vi "Dashboard Main.vi"() -> ()   [LabVIEW 2015]
uses:
  <vilib>/Utility/miscctls.llb/LVRowAndColumnTypeDef.ctl
  <vilib>/event_ctls.llb/eventvkey.ctl
  <vilib>/Rock Robotics/WPI/Dashboard/WPI_DashboardLogging Global.vi
  <vilib>/Rock Robotics/Network Tables/NT Read Numeric Array.vi
  <vilib>/Rock Robotics/Network Tables/NT Write Boolean.vi
  <vilib>/Utility/config.llb/Write Key (String).vi
  <vilib>/Utility/config.llb/Write Key (I32).vi
  <vilib>/Utility/config.llb/NI_LVConfig.lvlib
panel:
  in  "TCP":refnum<k5>
  in  "Rec Mode":enum32{"Stop", "Record", "Playback"}(radio)
  in  "Vision":u16(ring)=2 items=["Camera Off", "USB Camera SW", "USB Camera HW", "IP Camera"]
  out "Camera IP":string
  out "Image Message":string="Timeout in Camera Communications"
  in  "Dashboard Tab":T1(tab)
  in  "Select Auto":string(combo)
  out "NT Connection":bool
  in  "Camera Settings":T2={"Frame Rate"=30, "Compression"=30, "Size"=1} {"Frame Rate" scale=1.0..30.0; "Size" items=["640x480", "320x240", "160x120"]}
  out "MotorChart R":cluster{"Numeric":dbl, "Numeric":dbl}(graph)
  out "MotorChart L":T3(graph)
  out "MotorSliders R":cluster{"MotorSlide1":dbl, "MotorSlide2":dbl} {"MotorSlide2" scale=-1.0..1.0 scale format="%#_2e"; "MotorSlide1" scale=-1.0..1.0 scale format="%#_2e"}
  out "MotorSliders L":T4 {"MotorSlide4 2" scale=0.0..14.0 scale format="%#_2e"; "MotorSlide2" scale=-1.0..1.0 scale format="%#_2e"; "MotorSlide1" scale=-1.0..1.0 scale format="%#_2e"}
  out "Gyro":dbl(knob) scale=0.0..360.0
  out "JS1 Z":dbl(slide) scale=-1.0..1.0 scale format="%#_2e"
  out "JS1 Graph":cluster{"X":dbl, "Y":dbl}[](graph)
  out "JS1 Buttons":T5
  out "JS2 Z":dbl(slide) scale=-1.0..1.0 scale format="%#_2e"
  out "JS2 Graph":cluster{"X":dbl, "Y":dbl}[](graph)
  out "JS2 Buttons":T5
  out "Mode":T6(ring)=enum."Auto Disabled"
  in  "DB Camera Config":bool
  out "fps":dbl format="%#.1g"
  out "Mbps":dbl format="%#.1g"
  out "Mbps LED":bool
  in  "Camera Switch":bool
  in  "DB/String 9":string
  in  "DB/String 8":string
  in  "DB/String 7":string
  in  "DB/String 6":string
  in  "DB/String 5":string
  in  "DB/String 4":string
  in  "DB/String 3":string
  in  "DB/String 2":string
  in  "DB/String 1":string
  in  "DB/String 0":string
  in  "DB/Slider 0":dbl(slide) scale=0.0..5.0
  in  "DB/Slider 1":dbl(slide) scale=0.0..5.0
  in  "DB/Slider 2":dbl(slide) scale=0.0..5.0
  in  "DB/Slider 3":dbl(slide) scale=0.0..5.0
  out "DB/LED 3":bool
  out "DB/LED 2":bool
  out "DB/LED 1":bool
  out "DB/LED 0":bool
  in  "DB/Button 3":bool
  in  "DB/Button 2":bool
  in  "DB/Button 1":bool
  in  "DB/Button 0":bool caption="New Name"
  in  "Test Slider":dbl(slide) scale=0.0..100.0 scale format="%#_3g"
  in  "On/Off":bool caption="Solenoid"
  in  "Test Name":u16(ring) items=["Select the test to run..."]
  in  "Test Tree":string(tree)
  in  "Motor":cluster{"Value":dbl, "Enable":bool} {"Value" scale=-1.0..1.0 scale format="%#_3g"}
  out "Progress":T7 {"Test Progress" scale=0.0..100.0}
  in  "Rev/Fwd":cluster{"Forward":bool, "Reverse":bool}
  in  "Test Ring":u16(ring) items=["Monochrome", "Color"]
  out "Cmd Status":string
  in  "Execute Command":bool
  in  "Command Params":string[][](table)
  in  "Command Selection":i32(listbox)
  in  "CheckList":i32(listbox)
  out "Tree":string(tree)
  out "Camera Image":T8(plugin-control)
  out "Background":bool
  # "Left"
  # "Front"
  # "Right"
  # "Battery"
  # "This tab is a great place for autonomous settings and robot-specific values.\nPlace controls and indicators inside this tab and match name to\nDashboard Variables on robot. You can also delete this comment."
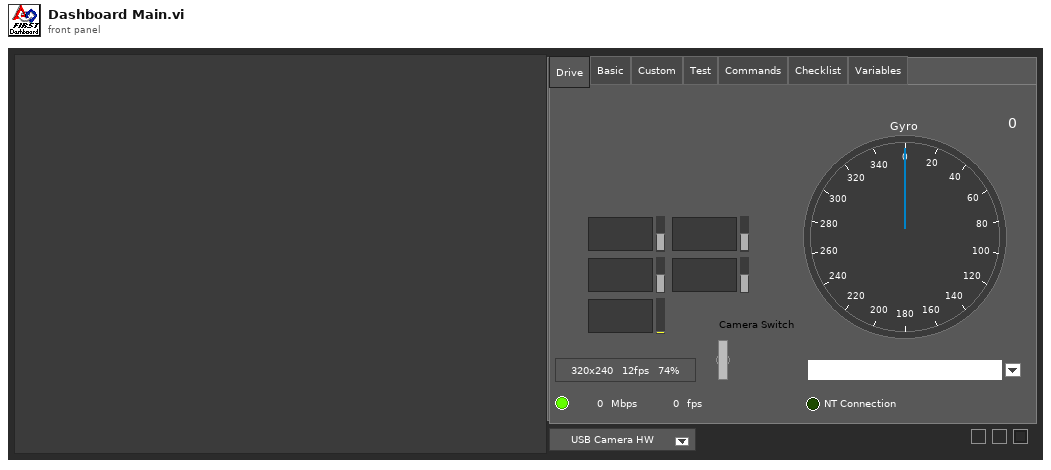
[diagram p1: front panel]
types:
  T1 = enum32{"Drive", "Basic", "Custom", "Test", "Commands", "Checklist", "Variables"}
  T2 = cluster{"Frame Rate":i32, "Compression":i32, "Size":u16}
  T3 = cluster{"Numeric":dbl, "Numeric":dbl, "Battery V":dbl}
  T4 = cluster{"MotorSlide1":dbl, "MotorSlide2":dbl, "MotorSlide4 2":dbl}
  T5 = cluster{bool, bool, bool, bool, bool, bool, bool, bool, bool, bool, bool, bool}
  T6 = enum8{"Tele-Op Disabled", "Tele-Op Enabled", "Auto Disabled", "Auto Enabled", "Test Disabled", "Test Enabled", "Disconnected", "No Code", "E-Stop"}
  T7 = cluster{"Test Progress":u8, "Test Progress Text":string}
  T8 = typedef "IMAQ Image.ctl" = refnum<image>
  T9 = cluster{"IDs":cluster{"RPC field ID":u16, "Unique ID":u16}, "String":string}
  T10 = enum32{"Drive", "Basic", "Custom", "Test", "Checklist", "Variables"}
  T11 = typedef "Image Type" = u32
  T12 = cluster{"Camera Image":refnum<vi>, "Dashboard Tab":refnum<vi>, "Background":refnum<vi>, "Vision":refnum<vi>, "Rec Mode":refnum<vi>, "Test Slider":refnum<vi>, "On/Off ":refnum<vi>, "Test Ring":refnum<vi>, "Rev/Fwd":refnum<vi>, "Test Name":refnum<vi>, "Motor":refnum<vi>, "Progress":refnum<vi>, "CheckList":refnum<vi>, "Tree":refnum<vi>, "Test Tree":refnum<vi>, "Command Params":refnum<vi>, "Command Selection":refnum<vi>, "Execute Command":refnum<vi>, "Cmd Status":refnum<vi>}
  T13 = cluster{"Error Strings":string, "Disable Counts":cluster{u16, u16}, "Rail Faults":cluster{u16, u16, u16}, "Robot IP":string, "DB Mode":u8, "Event Info":cluster{"Name":string, "Type":u8, "Number":u16, "Replay":u8}, "Camera Addr":string}
  T14 = cluster{"Storage":cluster{"Disk Free":u64, "RAM Block":u32, "RAM free":u32}, "CPU Utilization":cluster{"CPU % ISR":sgl, "CPU % Time Crit":sgl, "CPU % Timed Str":sgl, "CPU % High":sgl, "CPU % Above":sgl, "CPU % Normal":sgl, "CPU % Low":sgl}, "CAN":cluster{"% Bus Utilization":sgl, "Bus Off Cnt":u32, "TX_FIFO Full Cnt":u32, "Receive Error Cnt":u8, "Transmit Error Cnt":u8}, "HID":cluster{"HID Outputs":u32, "Rumble Low":u16, "Rumble High":u16}[]}
  T15 = cluster{"Status bits":cluster{"Test Mode":bool, "Autonomous":bool, "Enabled":bool, "Code Start":bool, "Brownout":bool, "Reserved 2":bool, "Reserved 3":bool, "E-Stop":bool}, "Code Trace":cluster{"Disabled":bool, "TeleOp":bool, "Auto":bool, "Test":bool}, "Controller Type":enum16{"unknown", "cRIO", "roboRio"}, "Code?":enum16{"unknown", "noCode", "code"}, "Battery V":dbl}
  T16 = cluster{"Control Bits":cluster{"TestMode":bool, "Autonomous":bool, "Enabled":bool, "FMS Present":bool, bool, bool, bool, "E-Stop":bool}, "Team Station ":u8, "Countdown":sgl, "Joystick Values":cluster{"Axes":dbl[], "Buttons":bool[], "POVs":i16[]}[]}
  T17 = cluster{"Axes":dbl[], "Buttons":bool[], "POVs":i16[]}[]
  T18 = cluster{"Axes":dbl[], "Buttons":bool[], "POVs":i16[]}
  T19 = cluster{"Buttons[0]":bool, "Buttons[1]":bool, "Buttons[2]":bool, "Buttons[3]":bool, "Buttons[4]":bool, "Buttons[5]":bool, "Buttons[6]":bool, "Buttons[7]":bool, "Buttons[8]":bool, "Buttons[9]":bool, "Buttons[10]":bool, "Buttons[11]":bool}
  T20 = typedef "NI_LVConfig.lvlib/Config Data RefNum.ctl" = refnum<k1>
  T21 = cluster{"Operation":enum16{"Update", "Clear"}, "Color Box":u32}[]
  T22 = typedef "eventvkey.ctl" = enum16{"ASCII", "Enter", "Return", "Shift", "Ctrl", "Alt", "Cmd", "Opt", "Caps", "NumLock", "Clear", "Break", "Up", "Down", "Left", "Right", "Insert", "Delete", "Home", "End", "PageUp", "PageDown", "Escape", "Help", "Pause", "ScrollLock", "F1", "F2", "F3", "F4", "F5", "F6", "F7", "F8", "F9", "F10", "F11", "F12", "F13", "F14", "F15", "F16", "F17", "F18", "F19", "F20", "F21", "F22", "F23", "F24", "Play", "VolumeUp", "VolumeDown", "Mute", "Two Byte Char"}
  T23 = cluster{"Image Size":bool, "Image Type":bool, "Pixel Value":bool, "ROI Information":bool, "Zoom Factor":bool}
  T24 = enum8{"Enabled", "Disabled", "Disabled and Grayed Out"}
  T25 = cluster{"Operation":enum16{"Update", "Clear"}, "Color Box":u32}
  T26 = typedef "LVRowAndColumnTypeDef.ctl" = cluster{"Row":i32, "Column":i32}
  T27 = cluster{"Shift":bool, "Ctrl":bool, "Alt":bool, "Cmd":bool, "Opt":bool}
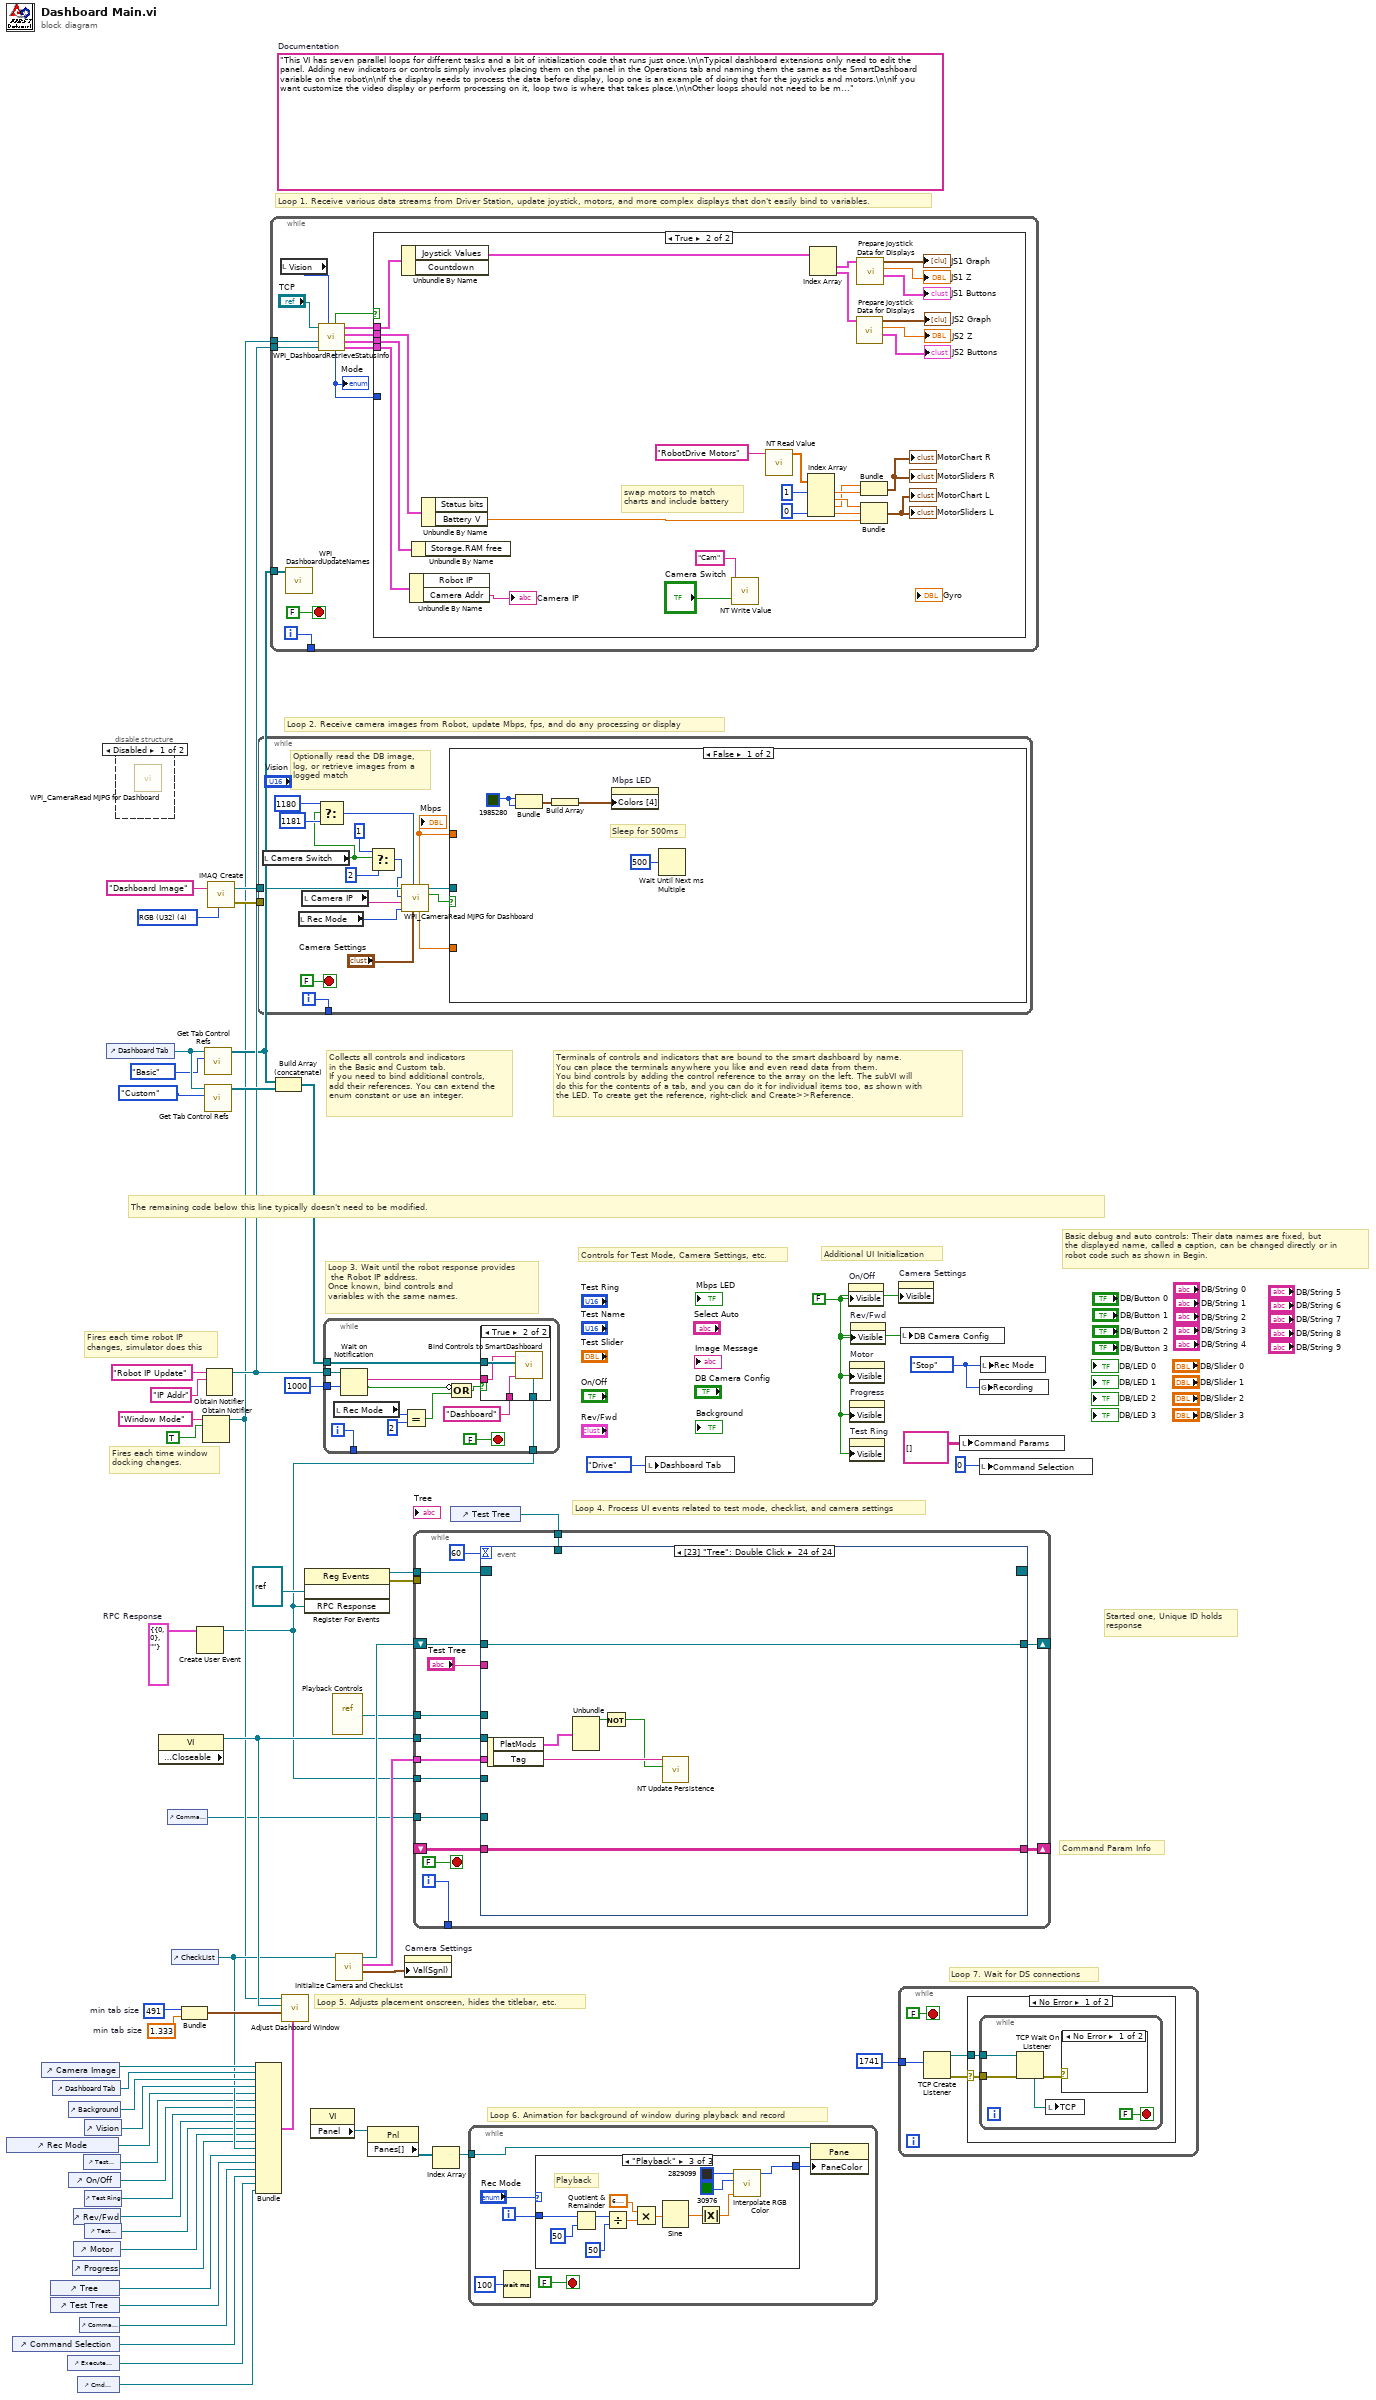
[diagram p0: block diagram]
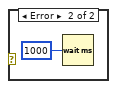
[diagram p3: hidden frame]
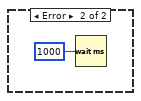
[diagram p4: hidden frame]
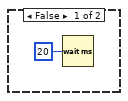
[diagram p5: hidden frame]
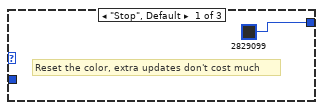
[diagram p6: hidden frame]
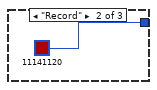
[diagram p7: hidden frame]
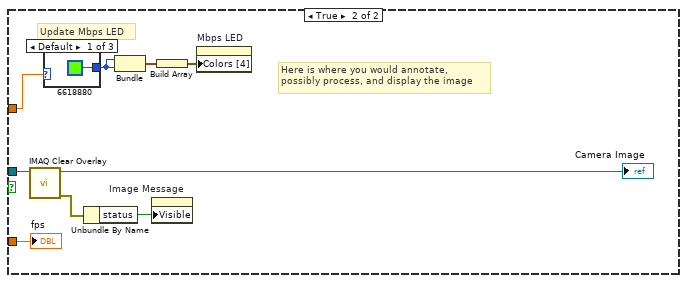
[diagram p9: hidden frame]
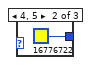
[diagram p10: hidden frame]
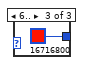
[diagram p11: hidden frame]
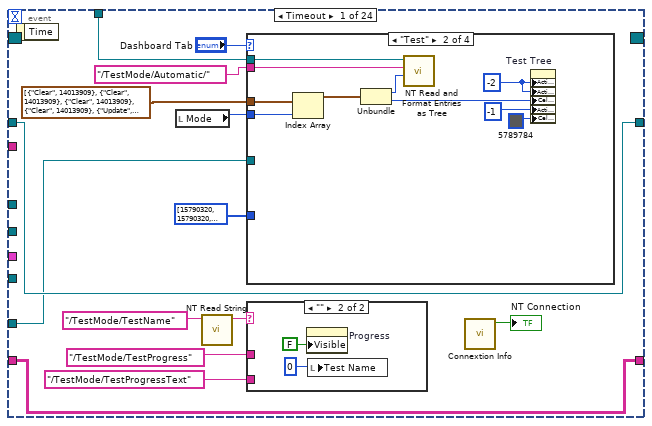
[diagram p12: hidden frame]
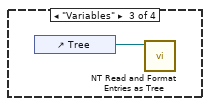
[diagram p14: hidden frame]
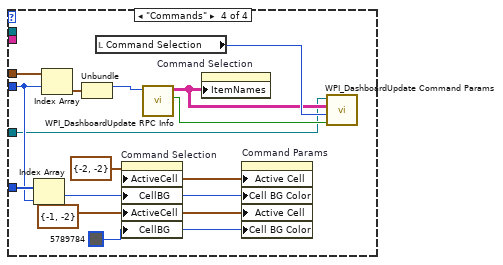
[diagram p15: hidden frame]
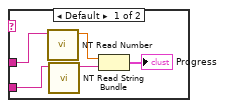
[diagram p16: hidden frame]
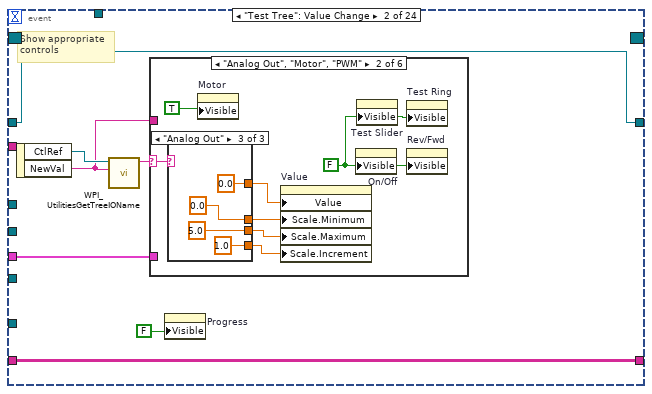
[diagram p17: hidden frame]
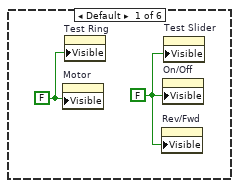
[diagram p18: hidden frame]
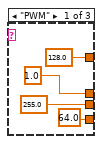
[diagram p19: hidden frame]
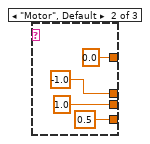
[diagram p20: hidden frame]
diagram:
  w7 = T9 {"IDs"={"RPC field ID"=0, "Unique ID"=0}, "String"=""}  # RPC Response
  w33 = 491  # min tab size
  w32 = 1.333  # min tab size
  w41 = enum32{"Stop", "Record", "Playback"}."Stop" ("Rec Mode")
  w15 = FALSE ("Visible")
  (unwired) "This VI has seven parallel loops for different tasks and a bit of initialization code that runs just once.\n\nTypical dashboard extensions only need to edit the panel. Adding new indicators or controls simply involves placing them on the panel in the Operations tab and naming them the same as the SmartDashboard variable on the robot\n\nIf the display needs to process the data before display, loop one is an example of doing that for the joysticks and motors.\n\nIf you want customize the video display or perform processing on it, loop two is where that takes place.\n\nOther loops should not need to be modified. They are pretty standard, and document the task they perform."  # Documentation
  w61 = T11 4 items=["Grayscale (U8)", "Grayscale (I16)", "Grayscale (SGL)", "Complex (CSG)", "RGB (U32)", "HSL (U32)", "RGB (U64)"] ("Image Type")
  # "Command Param Info"
  # "Started one, Unique ID holds\nresponse"
  # "Loop 7. Wait for DS connections"
  # "Basic debug and auto controls: Their data names are fixed, but\nthe displayed name, called a caption, can be changed directly or in\nrobot code such as shown in Begin."
  # "Controls for Test Mode, Camera Settings, etc."
  # "Additional UI Initialization"
  # "Loop 6. Animation for background of window during playback and record"
  # "Fires each time robot IP\nchanges, simulator does this"
  # "Fires each time window\ndocking changes."
  # "Collects all controls and indicators\nin the Basic and Custom tab.\nIf you need to bind additional controls,\nadd their references. You can extend the\nenum constant or use an integer."
  # "The remaining code below this line typically doesn't need to be modified."
  # "Loop 4. Process UI events related to test mode, checklist, and camera settings"
  # "Terminals of controls and indicators that are bound to the smart dashboard by name.\nYou can place the terminals anywhere you like and even read data from them.\nYou bind controls by adding the control reference to the array on the left. The subVI will\ndo this for the contents of a tab, and you can do it for individual items too, as shown with\nthe LED. To create get the reference, right-click and Create>>Reference."
  # "Loop 3. Wait until the robot response provides\n the Robot IP address.\nOnce known, bind controls and\nvariables with the same names."
  # "Loop 5. Adjusts placement onscreen, hides the titlebar, etc."
  # "Loop 1. Receive various data streams from Driver Station, update joystick, motors, and more complex displays that don't easily bind to variables."
  # "Loop 2. Receive camera images from Robot, update Mbps, fps, and do any processing or display"
  n1 = control-ref of="Rec Mode"() -> (w21:refnum<vi>)
  n2 = control-ref of="Command Selection"() -> (w6:refnum<vi>)
  n3 = control-ref of="Camera Image"() -> (w36:refnum<vi>)
  n4 = control-ref of="Tree"() -> (w25:refnum<vi>)
  n5 = control-ref of="Test Tree"() -> (w24:refnum<vi>)
  n6 = control-ref of="Dashboard Tab"() -> (w35:refnum<vi>)
  n7 = control-ref of="Execute Command"() -> (w8:refnum<vi>)
  n8 = control-ref of="Background"() -> (w30:refnum<vi>)
  n9 = control-ref of="On/Off"() -> (w19:refnum<vi>)
  n10 = control-ref of="Progress"() -> (w16:refnum<vi>)
  n11 = control-ref of="Rev/Fwd"() -> (w17:refnum<vi>)
  n12 = control-ref of="Motor"() -> (w22:refnum<vi>)
  n13 = control-ref of="Cmd Status"() -> (w2:refnum<vi>)
  n14 = control-ref of="Command Params"() -> (w9:refnum<vi>)
  n15 = control-ref of="Test Slider"() -> (w20:refnum<vi>)
  n16 = control-ref of="Vision"() -> (w34:refnum<vi>)
  n17 = control-ref of="Test Ring"() -> (w18:refnum<vi>)
  n18 = control-ref of="Test Name"() -> (w23:refnum<vi>)
  n19 = control-ref of="Dashboard Tab"() -> (w39:refnum<vi>)
  n20 = disable-structure shown="Disabled" {
    frame Disabled {
      n21 = call <vilib>:"WPI_CameraRead MJPG for Dashboard.vi"() -> ()  [unwired: 8 in, 4 out]
    }
    frame Enabled {
    }
  }
  n22 = property class="VI" props=["Front Panel.Closeable"]() -> (reference out=w40:refnum<vi>)  [unwired: 2 in, 2 out]
  n23 = control-ref of="Command Params"() -> (w1:refnum<vi>)
  n24 = control-ref of="CheckList"() -> (w26:refnum<vi>)
  n25 = Bundle("min tab size"=w33, "min tab size"=w32) -> (w31:cluster{"min tab size":i32, "min tab size":dbl})  [unwired: 1 in]
  n26 = Create User Event(user event datatype=w7) -> (user event=w3:refnum<user-event>)  [unwired: 1 in, 1 out]
  n27 = Obtain Notifier(name (unnamed)="Window Mode", notification data type=TRUE) -> (notifier out=w12:refnum<notifier>)  [unwired: 2 in, 2 out]
  n28 = call <vilib>:"Get Tab Control Refs.vi"("Page Index"=T10."Basic" ("Dashboard Tab"), "TabControl in"=w39) -> ("ControlsOnPage"=w13:refnum<vi>[])  [unwired: 9 in]
  n29 = call <vilib>:"Get Tab Control Refs.vi"("Page Index"=T10."Custom" ("Dashboard Tab"), "TabControl in"=w39) -> ("ControlsOnPage"=w38:refnum<vi>[])  [unwired: 9 in]
  n30 = Obtain Notifier(name (unnamed)="Robot IP Update", notification data type="IP Addr" ("name (unnamed)")) -> (notifier out=w14:refnum<notifier>)  [unwired: 2 in, 2 out]
  n31 = call "IMAQ Create"("Image Name"="Dashboard Image", "Image Type"=w61) -> ("New Image"=w59:T8, "error out"=w58:errorcluster)  [unwired: 2 in, 1 out]
  n32 = Bundle("Camera Image"=w36, "Dashboard Tab"=w35, "Background"=w30, "Vision"=w34, "Rec Mode"=w21, "Test Slider"=w20, "On/Off"=w19, "Test Ring"=w18, "Rev/Fwd"=w17, "Test Name"=w23, "Motor"=w22, "Progress"=w16, "CheckList"=w26, "Tree"=w25, "Test Tree"=w24, "Command Params"=w9, "Command Selection"=w6, "Execute Command"=w8, "Cmd Status"=w2) -> (w27:T12)  [unwired: 1 in]
  n33 = while {
    tunnel: w59 -> [w76]
    tunnel: w58 -> [_]
    tunnel: [w77] -> _
    i -> [w77]
    stop <- FALSE stop-if-true
    # "Optionally read the DB image,\nlog, or retrieve images from a\nlogged match"
    n34 = local read "Camera Switch"() -> (w65:bool)
    n35 = local read "Rec Mode"() -> (w71:enum32{"Stop", "Record", "Playback"})
    n36 = local read "Camera IP"() -> (w70:string)
    n37 = Select(t=1180, s=w65, f=1181) -> (s? t:f=w67:i32)
    n38 = Select(t=1, s=w65, f=2) -> (s? t:f=w62:i32)
    n39 = call <vilib>:"WPI_CameraRead MJPG for Dashboard.vi"("Camera Settings"="Camera Settings", "Camera Port"=w67, "Rec Mode"=w71, "Camera IP"=w70, "Camera Mode"=w62, "Refnum in"=w76) -> ("Active"=w74:bool, "Refnum out"=w75:T8, "FPS"=w73:dbl, "Bandwidth (Mbps)"=w69:dbl)  [unwired: 2 in]
    "Mbps" <- w69
    n40 = case shown="False" w74 {
      tunnel: w75 -> [_ w86]
      tunnel: w69 -> [_ w85]
      tunnel: w73 -> [_ w83]
      frame False {
        w79 = u32 1985280 ("Color Box")
        # "Sleep for 500ms"
        n41 = Bundle("Color Box"=w79, "Color Box"=w79) -> (w81:cluster{"Color Box":u32, "Color Box":u32})  [unwired: 1 out]
        n42 = Build Array(w81) -> (w80:cluster{"Color Box":u32, "Color Box":u32}[])
        n43 = property on="Mbps LED" class="Bool (strict)"("Colors [4]"=w80) -> ()  [unwired: 2 in, 2 out]
        n44 = Wait Until Next ms Multiple(millisecond multiple=u32 500) -> ()  [unwired: 1 out]
      }
      frame True {
        # "Here is where you would annotate,\npossibly process, and display the image"
        # "Update Mbps LED"
        n45 = call "IMAQ Clear Overlay"("Image"=w86) -> ("error out"=w90:errorcluster, "Image Out"=→"Camera Image":T8)  [unwired: 2 in, 7 out]
        n46 = case shown="Default" w85 {
          tunnel: [u32 6618880 ("Color Box") u32 16776722 ("Color Box") u32 16716800 ("Color Box")] -> w87
          frame Default {
          }
          frame 4, 5 {
          }
          frame 6.. {
          }
        }
        n47 = Unbundle By Name(w90) -> ("status"=w91:bool)
        n48 = Bundle("Color Box"=w87, "Color Box"=w87) -> (w89:cluster{"Color Box":u32, "Color Box":u32})  [unwired: 1 out]
        n49 = property on="Image Message" class="Str"("Visible"=w91) -> ()  [unwired: 2 in, 2 out]
        n50 = Build Array(w89) -> (w88:cluster{"Color Box":u32, "Color Box":u32}[])
        n51 = property on="Mbps LED" class="Bool (strict)"("Colors [4]"=w88) -> ()  [unwired: 2 in, 2 out]
        "fps" <- w83
      }
    }
  }
  n52 = while {
    tunnel: [w106] -> _
    tunnel: w14 -> [w100]
    tunnel: w13 -> [w99]
    tunnel: w12 -> [w95]
    i -> [w106]
    stop <- FALSE stop-if-true
    n53 = local read "Vision"() -> (w97:u16)
    n54 = call <vilib>:"WPI_DashboardUpdateNames.vi"("Controls on Tab"=w99) -> ()  [unwired: 11 in]
    n55 = call <vilib>:"WPI_DashboardRetrieveStatusInfo.vi"("Vision"=w97, "Binding Refnum"=w100, "Window Mode Notifier"=w95, "TCP Cnx"="TCP") -> ("Power and Errors"=w101:T13, "Robot Metrics"=w104:T14, "Status Info"=w105:T15, "Control Info"=w102:T16, "Robot Mode"=w98:T6, "Process?"=w103:bool)  [unwired: 2 in]
    "Mode" <- w98
    n56 = case shown="True" w103 {
      tunnel: w105 -> [_ w135]
      tunnel: w104 -> [_ w134]
      tunnel: w102 -> [_ w133]
      tunnel: w101 -> [_ w132]
      tunnel: w98 -> [_ _]
      frame False {
        n57 = Wait (ms)(milliseconds to wait=u32 20) -> ()  [unwired: 1 out]
      }
      frame True {
        # "swap motors to match\ncharts and include battery"
        n58 = Unbundle By Name(w133) -> ("Joystick Values"=w122:T17)  [unwired: 1 out]
        n59 = Unbundle By Name(w132) -> ("Camera Addr"=→"Camera IP":string)  [unwired: 1 out]
        n60 = Unbundle By Name(w134) -> ()  [unwired: 1 out]
        n61 = Unbundle By Name(w135) -> ("Battery V"=w123:dbl)  [unwired: 1 out]
        n62 = call-poly <vilib>:"NT Write Value.vi"("Boolean"="Camera Switch", "Name"="Cam") -> ()  [unwired: 9 in, 1 out]
        n63 = call-poly <vilib>:"NT Read Value.vi"("Name"="RobotDrive Motors") -> ("Numeric Array"=w111:dbl[])  [unwired: 9 in, 1 out]
        n64 = Index Array(array=w111, index #1=1, index #4=0) -> (element #1=w127:dbl, element #2=w128:dbl, element #3=w126:dbl, element #4=w131:dbl)  [unwired: 2 in]
        n65 = Index Array(array=w122) -> (element #1=w121:T18, element #2=w116:T18)  [unwired: 2 in]
        n66 = call "Prepare Joystick Data for Displays.vi"("Joystick Values"=w116) -> ("Buttons"=→"JS2 Buttons":T19, "Z Axis"=→"JS2 Z":dbl, "Cartesian Data"=→"JS2 Graph":cluster{"X axis":dbl, "X axis":dbl}[])  [unwired: 8 in]
        n67 = call "Prepare Joystick Data for Displays.vi"("Joystick Values"=w121) -> ("Buttons"=→"JS1 Buttons":T19, "Z Axis"=→"JS1 Z":dbl, "Cartesian Data"=→"JS1 Graph":cluster{"X axis":dbl, "X axis":dbl}[])  [unwired: 8 in]
        n68 = Bundle("Numeric"=w126, "Numeric"=w127) -> (→"MotorChart R" →"MotorSliders R":cluster{"Numeric":dbl, "Numeric":dbl})  [unwired: 1 in]
        n69 = Bundle("Numeric"=w128, "Numeric"=w131, "Battery V"=w123) -> (→"MotorChart L" →"MotorSliders L":T3)  [unwired: 1 in]
      }
    }
  }
  n70 = Build Array (concatenate)(w13, w38) -> (w37:refnum<vi>[])
  n71 = call "Adjust Dashboard Window.vi"("Sizing Refnums"=w27, "Size Constraints"=w31, "VI"=w40, "WIn Mode"=w12) -> ()  [unwired: 8 in]
  n72 = register-events(refnum<vi> refnum, w3) -> (reference out=w45:refnum<event-registration>, error out=w44:errorcluster)  [unwired: 2 in]
  n73 = property class="VI"() -> ("Panel"=w48:refnum<vi>)  [unwired: 2 in, 2 out]
  n74 = while {
    tunnel: w37 -> [w148]
    tunnel: w14 -> [w146]
    tunnel: [w144] -> _
    tunnel: u32 1000 ("milliseconds to wait") -> [w143]
    tunnel: w3 -> [w136]
    i -> [w144]
    stop <- FALSE stop-if-true
    n75 = local read "Rec Mode"() -> (w139:enum32{"Stop", "Record", "Playback"})
    n76 = Wait on Notification(notifier=w146, timeout in ms (-1)=w143) -> (notification=w145:string, timed out?=w141:bool)  [unwired: 2 in, 2 out]
    n77 = Equal?(x=w139, y=u16 2 ("Rec Mode")) -> (x = y?=w140:bool)
    n78 = Compound Arithmetic op=OR(invert w141, w140) -> (w142:bool)
    n79 = case shown="True" w142 {
      tunnel: w148 -> [_ w152]
      tunnel: w145 -> [_ w151]
      tunnel: "Dashboard" -> [_ w150]
      tunnel: w136 -> [_ w149]
      frame False {
      }
      frame True {
        n80 = call <vilib>:"Bind Controls to SmartDashboard.vi"("RPC ref"=w149, "Client Name"=w150, "Bound Control Refs"=w152, "Server IP Address"=w151) -> ()  [unwired: 8 in]
      }
    }
  }
  n81 = vi-ref "Playback Controls.vi"() -> (w46:refnum<vi>)
  n82 = call "Initialize Camera and CheckList.vi"("ListBox in"=w26) -> ("Cluster"=w52:cluster{"value":i32, "value":i32, "index":i32}, "Array"=w53:cluster{string[]}[], "File Refnum"=w51:T20)  [unwired: 8 in]
  n83 = property class="Pnl"(reference=w48) -> ("Panes[]"=w49:refnum<vi>[])  [unwired: 1 in, 2 out]
  n84 = property on="Camera Settings" class="Clust (strict)"("Val(Sgnl)"=w52) -> ()  [unwired: 2 in, 2 out]
  n85 = Index Array(array=w49) -> (element=w47:refnum<vi>)  [unwired: 1 in]
  n86 = control-ref of="Test Tree"() -> (w50:refnum<vi>)
  n87 = while {
    tunnel: w53 -> [w164]
    shift-right: [w163] -> _
    shift-left: w51 -> [w162]
    tunnel: [w161] -> _
    tunnel: w50 -> [w160]
    tunnel: w46 -> [w159]
    tunnel: w45 -> [w158]
    tunnel: w44 -> [_]
    tunnel: w40 -> [w157]
    tunnel: w3 -> [w156]
    tunnel: w1 -> [w155]
    shift-right: [w154] -> _
    shift-left: _ -> [w153]
    i -> [w161]
    stop <- FALSE stop-if-true
    n88 = event shown="[23] \"Tree\": Double Click" {
      selector: w158 -> [_ _ _ _ _ _ _ _ _ _ _ _ _ _ _ _ _ _ _ _ _ _ _ _]
      dyn-events: [_ _ _ _ _ _ _ _ _ _ _ _ _ _ _ _ _ _ w473 _ _ _ _ _] -> _
      timeout: u32 60 ("milliseconds to wait") -> [_ _ _ _ _ _ _ _ _ _ _ _ _ _ _ _ _ _ _ _ _ _ _ _]
      tunnel: w160 -> [w177 _ _ _ _ _ _ _ _ _ _ _ _ _ _ _ _ _ _ _ _ _ _ _]
      tunnel: "Test Tree" -> [_ _ _ _ _ _ _ _ _ _ _ _ _ w436 w445 w448 w453 w462 _ _ _ _ _ _]
      tunnel: w164 -> [_ w215 _ _ _ _ _ _ _ _ _ w398 w429 _ _ _ _ _ _ _ _ _ _ _]
      tunnel: [w174 w214 w318 w324 w334 w338 w344 w356 w364 w370 w383 w397 w422 w435 w443 w447 w452 w461 w475 w491 w493 w501 w512 w517] -> w163
      tunnel: w162 -> [w174 w214 w318 w324 w334 w338 w344 w356 w364 w370 w383 w396 w422 w435 w443 w447 w452 w461 w475 w491 w493 w501 w512 w517]
      tunnel: w159 -> [_ _ _ _ _ _ _ _ _ _ _ _ _ _ _ _ _ _ w476 _ w496 _ _ _]
      tunnel: w157 -> [_ _ _ _ _ _ _ _ _ _ _ _ _ _ _ _ _ _ w471 _ _ _ _ _]
      tunnel: w156 -> [_ _ _ _ _ _ _ _ _ _ _ _ _ _ _ _ _ _ w467 _ _ _ _ _]
      tunnel: w155 -> [w169 _ _ _ _ _ w342 _ _ _ _ _ _ _ _ _ _ _ _ _ _ _ _ _]
      tunnel: [w168 w213 w317 w323 w333 w339 w340 w350 w361 w369 w382 w395 w421 w434 w442 w446 w451 w460 w466 w489 w492 w497 w505 w518] -> w154
      tunnel: w153 -> [w168 w213 w317 w323 w333 w339 w340 _ _ w369 w382 w395 w421 w434 w442 w446 w451 w460 w466 w489 w492 w497 w505 w518]
      event Timeout {
        n89 = event-data() -> ()  [unwired: 1 in, 1 out]
        n90 = local read "Mode"() -> (w171:T6)
        n91 = call <vilib>:"NT Read String.vi"("Name"="/TestMode/TestName") -> ("String"=w180:string)  [unwired: 9 in, 1 out]
        n92 = case shown="\"Test\"" "Dashboard Tab" {
          tunnel: w177 -> [_ w191 _ _]
          tunnel: "/TestMode/Automatic/" ("Name Pattern") -> [_ w190 _ _]
          tunnel: T21 [{"Operation"=enum."Clear", "Color Box"=14013909}, {"Operation"=enum."Clear", "Color Box"=14013909}, {"Operation"=enum."Clear", "Color Box"=14013909}, {"Operation"=enum."Clear", "Color Box"=14013909}, {"Operation"=enum."Update", "Color Box"=14013909}, {"Operation"=enum."Update", "Color Box"=16777215}, {"Operation"=enum."Clear", "Color Box"=14013909}, {"Operation"=enum."Clear", "Color Box"=14013909}, {"Operation"=enum."Clear", "Color Box"=14013909}] -> [_ w183 _ w200]
          tunnel: w171 -> [_ w182 _ w199]
          tunnel: u32[] [15790320, 15790320, 15790320, 15790320, 16777215, 16777215, 15790320, 15790320, 15790320] -> [_ _ _ w205]
          tunnel: w169 -> [_ _ _ w193]
          frame "Custom", Default {
          }
          frame "Test" {
            w189 = -2 ("Active Item:Row Number")
            n93 = Index Array(array=w183, index=w182) -> (element=w184:T25)
            n94 = Unbundle(w184) -> ("Operation"=w185:enum16{"Update", "Clear"}, "Color Box"=w186:u32)
            n95 = call <vilib>:"NT Read and Format Entries as Tree.vi"("Operation"=w185, "Name Pattern"=w190, "Tree Refnum"=w191) -> ()  [unwired: 7 in, 2 out]
            n96 = property on="Test Tree" class="Tree (strict)"("Active Item Row Number"=w189, "ActiveColNum"=w189, "CellBG"=w186, "Active Item Row Number"=-1 ("Active Item:Row Number"), "CellBG"=u32 5789784 ("Color Box")) -> ()  [unwired: 2 in, 2 out]
          }
          frame "Variables" {
            n97 = control-ref of="Tree"() -> (w192:refnum<vi>)
            n98 = call <vilib>:"NT Read and Format Entries as Tree.vi"("Tree Refnum"=w192) -> ()  [unwired: 9 in, 2 out]
          }
          frame "Commands" {
            w201 = u32 5789784 ("Color Box")
            w202 = T26 {"Row"=-1, "Column"=-2} ("Active Cell:Active Cell")
            w204 = T26 {"Row"=-2, "Column"=-2} ("Active Cell:Active Cell")
            n99 = Index Array(array=w205, index=w199) -> (element=w203:u32)
            n100 = Index Array(array=w200, index=w199) -> (element=w198:T25)
            n101 = Unbundle(w198) -> ("Operation"=w197:enum16{"Update", "Clear"})  [unwired: 1 out]
            n102 = local read "Command Selection"() -> (w196:i32)
            n103 = property on="Command Selection" class="MCListbox (strict)"("ActiveCell"=w204, "CellBG"=w203, "ActiveCell"=w202, "CellBG"=w201) -> ()  [unwired: 2 in, 2 out]
            n104 = call <vilib>:"WPI_DashboardUpdate RPC Info.vi"("Operation"=w197) -> ("update"=w195:bool, "commands"=w194:string[][])  [unwired: 9 in]
            n105 = property on="Command Selection" class="MCListbox (strict)"("ItemNames"=w194) -> ()  [unwired: 2 in, 2 out]
            n106 = property on="Command Params" class="Tbl (strict)"("Active Cell"=w204, "Cell BG Color"=w203, "Active Cell"=w202, "Cell BG Color"=w201) -> ()  [unwired: 2 in, 2 out]
            n107 = call <vilib>:"WPI_DashboardUpdate Command Params.vi"("Update"=w195, "NewVal"=w196, "Commands"=w194, "Param Tbl"=w193) -> ()  [unwired: 7 in, 1 out]
          }
        }
        n108 = case shown="\"\"" w180 {
          tunnel: "/TestMode/TestProgress" ("Name") -> [w207 _]
          tunnel: "/TestMode/TestProgressText" ("Name") -> [w206 _]
          frame Default {
            n109 = call <vilib>:"NT Read Number.vi"("Name"=w207) -> ("Numeric"=w208:dbl)  [unwired: 9 in, 1 out]
            n110 = call <vilib>:"NT Read String.vi"("Name"=w206) -> ("String"=w209:string)  [unwired: 9 in, 1 out]
            n111 = Bundle("Numeric"=w208, "String"=w209) -> (→"Progress":cluster{"Numeric":dbl, "String":string})  [unwired: 1 in]
          }
          frame "" {
            n112 = property on="Progress" class="Clust (strict)"("Visible"=FALSE) -> ()  [unwired: 2 in, 2 out]
            n113 = local write "Test Name"(u16 0) -> ()
          }
        }
        n114 = call <vilib>:"Connextion Info.vi"() -> ("Connected"=→"NT Connection":bool)  [unwired: 10 in, 1 out]
      }
      event "Test Tree": Value Change {
        # "Show appropriate\ncontrols"
        n115 = event-data() -> ("CtlRef"=w218:refnum<vi>, "NewVal"=w216:string)  [unwired: 1 in]
        n116 = call <vilib>:"WPI_UtilitiesGetTreeIOName.vi"("NewVal"=w216, "TreeControl in"=w218) -> ("I/O Name"=w219:string)  [unwired: 9 in]
        n117 = case shown="\"Analog Out\", \"Motor\", \"PWM\"" w219 {
          selector: w219 -> [_ w226 _ w248 w257 _]
          tunnel: w216 -> [_ _ w245 w247 _ w264]
          tunnel: w215 -> [_ _ _ _ _ w263]
          frame Default {
            w221 = FALSE ("Visible")
            w220 = FALSE ("Visible")
            n118 = property on="Motor" class="Clust (strict)"("Visible"=w220) -> ()  [unwired: 2 in, 2 out]
            n119 = property on="Test Ring" class="Ring (strict)"("Visible"=w220) -> ()  [unwired: 2 in, 2 out]
            n120 = property on="Rev/Fwd" class="Clust (strict)"("Visible"=w221) -> ()  [unwired: 2 in, 2 out]
            n121 = property on="On/Off" class="Bool (strict)"("Visible"=w221) -> ()  [unwired: 2 in, 2 out]
            n122 = property on="Test Slider" class="Slide (strict)"("Visible"=w221) -> ()  [unwired: 2 in, 2 out]
          }
          frame "Analog Out", "Motor", "PWM" {
            w227 = FALSE ("Visible")
            n123 = case shown="\"Analog Out\"" w226 {
              tunnel: [1.0 ("Value") -1.0 ("Value") 0.0 ("Value")] -> w225
              tunnel: [255.0 ("Value") 1.0 ("Value") 5.0 ("Value")] -> w224
              tunnel: [128.0 ("Value") 0.0 ("Value") 0.0 ("Value")] -> w223
              tunnel: [64.0 ("Value") 0.5 ("Value") 1.0 ("Value")] -> w222
              frame "PWM" {
              }
              frame "Motor", Default {
              }
              frame "Analog Out" {
              }
            }
            n124 = property on="Motor" class="Clust (strict)"("Visible"=TRUE) -> ()  [unwired: 2 in, 2 out]
            n125 = property on="Value" class="Slide (strict)"("Value"=w223, "Scale.Minimum"=w225, "Scale.Maximum"=w224, "Scale.Increment"=w222) -> ()  [unwired: 2 in, 2 out]
            n126 = property on="On/Off" class="Bool (strict)"("Visible"=w227) -> ()  [unwired: 2 in, 2 out]
            n127 = property on="Test Slider" class="Slide (strict)"("Visible"=w227) -> ()  [unwired: 2 in, 2 out]
            n128 = property on="Test Ring" class="Ring (strict)"("Visible"=w227) -> ()  [unwired: 2 in, 2 out]
            n129 = property on="Rev/Fwd" class="Clust (strict)"("Visible"=w227) -> ()  [unwired: 2 in, 2 out]
          }
          frame "Servo" {
            w243 = FALSE ("Visible")
            n130 = call <vilib>:"NT Read Number.vi"("Name"=w245) -> ("Numeric"=w244:dbl)  [unwired: 9 in, 1 out]
            n131 = property on="Test Slider" class="Slide (strict)"("Visible"=TRUE, "Scale.Maximum"=170.0 ("Scale.Range:Maximum")) -> ()  [unwired: 2 in, 2 out]
            n132 = local write "Test Slider"(w244) -> ()
            n133 = property on="Motor" class="Clust (strict)"("Visible"=w243) -> ()  [unwired: 2 in, 2 out]
            n134 = property on="Rev/Fwd" class="Clust (strict)"("Visible"=w243) -> ()  [unwired: 2 in, 2 out]
            n135 = property on="On/Off" class="Bool (strict)"("Visible"=w243) -> ()  [unwired: 2 in, 2 out]
            n136 = property on="Test Ring" class="Ring (strict)"("Visible"=w243) -> ()  [unwired: 2 in, 2 out]
          }
          frame "Relay", "Solenoid" {
            w246 = FALSE ("Visible")
            n137 = property on="Motor" class="Clust (strict)"("Visible"=w246) -> ()  [unwired: 2 in, 2 out]
            n138 = property on="Test Slider" class="Slide (strict)"("Visible"=w246) -> ()  [unwired: 2 in, 2 out]
            n139 = Search and Replace String(input string=w247, search string="/Value  **", replace string="/Direction") -> (result string=w253:string)  [unwired: 5 in, 3 out]
            n140 = property on="Test Ring" class="Ring (strict)"("Visible"=w246) -> ()  [unwired: 2 in, 2 out]
            n141 = call <vilib>:"NT Read String.vi"("Name"=w253) -> ("String"=w251:string)  [unwired: 9 in, 1 out]
            n142 = Equal?(x="Both directions", y=w251) -> (x = y?=w249:bool)
            n143 = Not(x=w249) -> (.not. x?=w250:bool)
            n144 = property on="Rev/Fwd" class="Clust (strict)"("Visible"=w249) -> ()  [unwired: 2 in, 2 out]
            n145 = property on="On/Off" class="Bool (strict)"("Visible"=w250, "Caption.Text"=w248) -> ()  [unwired: 2 in, 2 out]
          }
          frame "Compressor", "Digital Out" {
            w256 = FALSE ("Visible")
            # "Get direction and finish"
            n146 = property on="Motor" class="Clust (strict)"("Visible"=w256) -> ()  [unwired: 2 in, 2 out]
            n147 = property on="Test Slider" class="Slide (strict)"("Visible"=w256) -> ()  [unwired: 2 in, 2 out]
            n148 = property on="Test Ring" class="Ring (strict)"("Visible"=w256) -> ()  [unwired: 2 in, 2 out]
            n149 = property on="On/Off" class="Bool (strict)"("Visible"=TRUE, "Caption.Text"=w257) -> ()  [unwired: 2 in, 2 out]
            n150 = property on="Rev/Fwd" class="Clust (strict)"("Visible"=FALSE) -> ()  [unwired: 2 in, 2 out]
          }
          frame "Camera" {
            n151 = call <vilib>:"Get Last Path Segment.vi"("String in"=w264) -> ("String out"=w265:string)  [unwired: 10 in]
            n152 = property on="On/Off" class="Bool (strict)"("Visible"=FALSE) -> ()  [unwired: 2 in, 2 out]
            n153 = property on="Motor" class="Clust (strict)"("Visible"=FALSE) -> ()  [unwired: 2 in, 2 out]
            n154 = property on="Rev/Fwd" class="Clust (strict)"("Visible"=FALSE) -> ()  [unwired: 2 in, 2 out]
            n155 = case shown="\"White Balance  **\"" w265 {
              tunnel: w264 -> [w271 w280 w289 w298 w307 _ w313]
              tunnel: w263 -> [w269 w277 w286 w295 w304 _ _]
              frame "Size  **" {
                n156 = Index Array(array=w269) -> (element=w268:cluster{string[]})  [unwired: 1 in]
                n157 = call <vilib>:"NT Read String.vi"("Name"=w271) -> ("String"=w270:string)  [unwired: 9 in, 1 out]
                n158 = Unbundle(w268) -> (w266:string[])
                n159 = Match First String(2:w266, 3:w270) -> (0:w267:i32)  [unwired: 1 out]
                n160 = property on="Test Ring" class="Ring (strict)"("Value"=w267, "Strings []"=w266) -> ()  [unwired: 2 in, 2 out]
                n161 = property on="Test Ring" class="Ring (strict)"("Visible"=TRUE) -> ()  [unwired: 2 in, 2 out]
                n162 = property on="Test Slider" class="Slide (strict)"("Visible"=FALSE) -> ()  [unwired: 2 in, 2 out]
              }
              frame "White Balance  **" {
                n163 = Index Array(array=w277, index=1) -> (element=w278:cluster{string[]})
                n164 = call <vilib>:"NT Read String.vi"("Name"=w280) -> ("String"=w279:string)  [unwired: 9 in, 1 out]
                n165 = Unbundle(w278) -> (w275:string[])
                n166 = Match First String(2:w275, 3:w279) -> (0:w274:i32)  [unwired: 1 out]
                n167 = property on="Test Ring" class="Ring (strict)"("Value"=w274, "Strings []"=w275) -> ()  [unwired: 2 in, 2 out]
                n168 = property on="Test Ring" class="Ring (strict)"("Visible"=TRUE) -> ()  [unwired: 2 in, 2 out]
                n169 = property on="Test Slider" class="Slide (strict)"("Visible"=FALSE) -> ()  [unwired: 2 in, 2 out]
              }
              frame "Exposure  **" {
                n170 = Index Array(array=w286, index=2) -> (element=w287:cluster{string[]})
                n171 = call <vilib>:"NT Read String.vi"("Name"=w289) -> ("String"=w288:string)  [unwired: 9 in, 1 out]
                n172 = Unbundle(w287) -> (w283:string[])
                n173 = Match First String(2:w283, 3:w288) -> (0:w284:i32)  [unwired: 1 out]
                n174 = property on="Test Ring" class="Ring (strict)"("Value"=w284, "Strings []"=w283) -> ()  [unwired: 2 in, 2 out]
                n175 = property on="Test Ring" class="Ring (strict)"("Visible"=TRUE) -> ()  [unwired: 2 in, 2 out]
                n176 = property on="Test Slider" class="Slide (strict)"("Visible"=FALSE) -> ()  [unwired: 2 in, 2 out]
              }
              frame "Exposure Priority  **" {
                n177 = Index Array(array=w295, index=3) -> (element=w296:cluster{string[]})
                n178 = call <vilib>:"NT Read String.vi"("Name"=w298) -> ("String"=w297:string)  [unwired: 9 in, 1 out]
                n179 = Unbundle(w296) -> (w292:string[])
                n180 = Match First String(2:w292, 3:w297) -> (0:w293:i32)  [unwired: 1 out]
                n181 = property on="Test Ring" class="Ring (strict)"("Value"=w293, "Strings []"=w292) -> ()  [unwired: 2 in, 2 out]
                n182 = property on="Test Ring" class="Ring (strict)"("Visible"=TRUE) -> ()  [unwired: 2 in, 2 out]
                n183 = property on="Test Slider" class="Slide (strict)"("Visible"=FALSE) -> ()  [unwired: 2 in, 2 out]
              }
              frame "Color Enable  **" {
                n184 = Index Array(array=w304, index=4) -> (element=w305:cluster{string[]})
                n185 = call <vilib>:"NT Read String.vi"("Name"=w307) -> ("String"=w306:string)  [unwired: 9 in, 1 out]
                n186 = Unbundle(w305) -> (w301:string[])
                n187 = Match First String(2:w301, 3:w306) -> (0:w302:i32)  [unwired: 1 out]
                n188 = property on="Test Ring" class="Ring (strict)"("Value"=w302, "Strings []"=w301) -> ()  [unwired: 2 in, 2 out]
                n189 = property on="Test Ring" class="Ring (strict)"("Visible"=TRUE) -> ()  [unwired: 2 in, 2 out]
                n190 = property on="Test Slider" class="Slide (strict)"("Visible"=FALSE) -> ()  [unwired: 2 in, 2 out]
              }
              frame Default {
                n191 = property on="Test Ring" class="Ring (strict)"("Visible"=FALSE) -> ()  [unwired: 2 in, 2 out]
                n192 = property on="Test Slider" class="Slide (strict)"("Visible"=FALSE) -> ()  [unwired: 2 in, 2 out]
              }
              frame "Brightness  **", "Color Level  **", "Compression  **", "FPS  **", "Sharpness  **" {
                n193 = call <vilib>:"NT Read Number.vi"("Name"=w313) -> ("Numeric"=w312:dbl)  [unwired: 9 in, 1 out]
                n194 = local write "Test Slider"(w312) -> ()
                n195 = property on="Test Slider" class="Slide (strict)"("Visible"=TRUE, "Scale.Maximum"=100.0 ("Scale.Range:Maximum")) -> ()  [unwired: 2 in, 2 out]
                n196 = property on="Test Ring" class="Ring (strict)"("Visible"=FALSE) -> ()  [unwired: 2 in, 2 out]
              }
            }
          }
        }
        n197 = property on="Progress" class="Clust (strict)"("Visible"=FALSE) -> ()  [unwired: 2 in, 2 out]
      }
      event "Test Name": Mouse Enter {
        # "Populate the ring with the list of tests"
        n198 = event-data() -> ()  [unwired: 1 in, 1 out]
        n199 = call <vilib>:"NT Read String Array.vi"("Name"="/TestMode/TestList") -> ("String Array"=w322:string[])  [unwired: 9 in, 1 out]
        n200 = Build Array (concatenate)("Select the test to run...", w322) -> (w321:string[])
        n201 = property on="Test Name" class="Ring (strict)"("Strings []"=w321) -> ()  [unwired: 2 in, 2 out]
      }
      event "Test Name": Value Change {
        w325 = FALSE ("Visible")
        # "Tell the robot the test name to run"
        n202 = event-data() -> ("NewVal"=w329:u16)  [unwired: 1 in]
        n203 = property on="Test Name" class="Ring (strict)"() -> ("Strings []"=w330:string[])  [unwired: 2 in, 2 out]
        n204 = local write "Progress"(T7 {"Test Progress"=0, "Test Progress Text"=""} ("Progress")) -> ()
        n205 = Index Array(array=w330, index=w329) -> (element=w328:string)
        n206 = call <vilib>:"NT Write String.vi"("String"=w328, "Name"="/TestMode/TestName") -> ()  [unwired: 9 in, 1 out]
        n207 = property on="Progress" class="Clust (strict)"("Visible"=TRUE) -> ()  [unwired: 2 in, 2 out]
        n208 = property on="Motor" class="Clust (strict)"("Visible"=w325) -> ()  [unwired: 2 in, 2 out]
        n209 = property on="Test Slider" class="Slide (strict)"("Visible"=w325) -> ()  [unwired: 2 in, 2 out]
        n210 = property on="On/Off" class="Bool (strict)"("Visible"=w325) -> ()  [unwired: 2 in, 2 out]
        n211 = property on="Rev/Fwd" class="Clust (strict)"("Visible"=w325) -> ()  [unwired: 2 in, 2 out]
        n212 = property on="Test Ring" class="Ring (strict)"("Visible"=w325) -> ()  [unwired: 2 in, 2 out]
      }
      event "Select Auto": Mouse Enter {
        # "Populate the combo box with the list of autonomous options"
        n213 = event-data() -> ()  [unwired: 1 in, 1 out]
        n214 = call <vilib>:"NT Read String Array.vi"("Name"="Auto List") -> ("String Array"=w332:string[])  [unwired: 9 in, 1 out]
        n215 = property on="Select Auto" class="CmbBox"("Strings[]"=w332) -> ()  [unwired: 2 in, 2 out]
      }
      event "Select Auto": Value Change {
        # "User modified the Auto Selection. Write to NT variable so robot knows."
        n216 = event-data() -> ("NewVal"=w336:string)  [unwired: 1 in]
        n217 = call <vilib>:"NT Write String.vi"("String"=w336, "Name"="Auto Selector") -> ()  [unwired: 9 in, 1 out]
      }
      event "Command Selection": Value Change {
        # "Get the params and show in table"
        n218 = event-data() -> ("NewVal"=w343:i32)  [unwired: 1 in]
        n219 = property on="Command Selection" class="MCListbox (strict)"() -> ("ItemNames"=w341:string[][])  [unwired: 2 in, 2 out]
        n220 = call <vilib>:"WPI_DashboardUpdate Command Params.vi"("NewVal"=w343, "Commands"=w341, "Param Tbl"=w342) -> ()  [unwired: 8 in, 1 out]
      }
      event "Execute Command": Value Change {
        # "Started one, Unique ID holds\nresponse"
        n221 = event-data() -> ()  [unwired: 1 in, 1 out]
        n222 = property on="Command Selection" class="MCListbox (strict)"() -> ("ItemNames"=w355:string[][])  [unwired: 2 in, 2 out]
        n223 = Index Array(array=w355, index (row)="Command Selection", index (col)=0) -> (element=w353:string)
        n224 = call <vilib>:"Invoke Commands.vi"("Command Params"="Command Params", "Function Name"=w353) -> ("Params"=w349:u8, "Started"=w348:bool)  [unwired: 7 in, 1 out]
        n225 = Array Subset(array="Command Params", length (row)=w349) -> (w350:string[][])  [unwired: 3 in]
        n226 = Select(t="Executing" ("Cmd Status"), s=w348, f="" ("Cmd Status")) -> (s? t:f=→"Cmd Status":string)
      }
      event "Command Selection": Double Click {
        n227 = event-data() -> ("Row"=w365:i32)  [unwired: 1 in]
        n228 = property on="Command Selection" class="MCListbox (strict)"() -> ("ItemNames"=w368:string[][])  [unwired: 2 in, 2 out]
        n229 = local read "Command Params"() -> (w363:string[][])
        n230 = Index Array(array=w368, index (row)=w365, index (col)=0) -> (element=w366:string)
        n231 = call <vilib>:"Invoke Commands.vi"("Command Params"=w363, "Function Name"=w366) -> ("Params"=w362:u8, "Started"=w357:bool)  [unwired: 7 in, 1 out]
        n232 = Array Subset(array=w363, length (row)=w362) -> (w361:string[][])  [unwired: 3 in]
        n233 = Select(t="Executing" ("Cmd Status"), s=w357, f="" ("Cmd Status")) -> (s? t:f=w358:string)
        n234 = local write "Cmd Status"(w358) -> ()
      }
      event "CheckList": Double Click {
        # "Shift clears all"
        # "Update symbols on the listbox"
        n235 = event-data() -> ("PlatMods.Shift"=w371:bool, "Row"=w373:i32)  [unwired: 1 in]
        n236 = case shown="True" w371 {
          tunnel: w373 -> [w377 _]
          tunnel: 1 -> [w376 _]
          frame False {
            n237 = property on="CheckList" class="LstBox (strict)"() -> ("Item Symbols"=w375:i32[])  [unwired: 2 in, 2 out]
            n238 = Replace Array Subset(array=w375, new element=w376, index=w377) -> (w374:i32[])
            n239 = property on="CheckList" class="LstBox (strict)"("Item Symbols"=w374) -> ()  [unwired: 2 in, 2 out]
          }
          frame True {
            w378 = 0 ("Top Row")
            n240 = property on="CheckList" class="LstBox (strict)"() -> ("Number of Rows"=w380:u32)  [unwired: 2 in, 2 out]
            n241 = Initialize Array(0, w380) -> (w379:i32[])
            n242 = property on="CheckList" class="LstBox (strict)"("Top Row"=w378, "Value"=w378, "Item Symbols"=w379) -> ()  [unwired: 2 in, 2 out]
          }
        }
      }
      event "CheckList": Key Down {
        # "Update symbols on the listbox\nLeft and right keys check and uncheck"
        n243 = event-data() -> ("VKey"=w385:T22)  [unwired: 1 in]
        n244 = case shown="\"Left\", \"Right\"" w385 {
          selector: w385 -> [w390 _]
          tunnel: eventvkey."Left" ("VKey") -> [w388 _]
          frame "Left", "Right" {
            n245 = Equal?(x=w388, y=w390) -> (x = y?=w389:bool)
            n246 = Select(t=0, s=w389, f=1) -> (s? t:f=w391:i32)
            n247 = property on="CheckList" class="LstBox (strict)"() -> ("Item Symbols"=w394:i32[])  [unwired: 2 in, 2 out]
            n248 = Replace Array Subset(array=w394, new element=w391, index="CheckList") -> (w393:i32[])
            n249 = property on="CheckList" class="LstBox (strict)"("Item Symbols"=w393) -> ()  [unwired: 2 in, 2 out]
          }
          frame Default {
          }
        }
      }
      event "DB Camera Config": Value Change {
        # "Show or hide the cluster of controls, store in ini file"
        n250 = event-data() -> ("NewVal"=w399:bool)  [unwired: 1 in]
        n251 = case shown="False" w399 {
          tunnel: w398 -> [w408 _]
          tunnel: [w401 w419] -> w397
          tunnel: w396 -> [w400 w419]
          frame False {
            w415 = "Camera"
            w418 = FALSE ("Visible")
            n252 = local read "Camera Settings"() -> (w407:T2)
            n253 = Index Array(array=w408) -> (element=w411:cluster{string[]})  [unwired: 1 in]
            n254 = Unbundle(w407) -> ("Frame Rate"=w406:i32, "Compression"=w405:i32, "Size"=w409:u16)
            n255 = Unbundle(w411) -> (w410:string[])
            n256 = Index Array(array=w410, index=w409) -> (element=w404:string)
            n257 = call-poly <vilib>:"Write Key.vi"("section"=w415, "value"=w404, "key"="Size", "refnum"=w400) -> ("refnum out"=w417:T20)  [unwired: 2 in, 5 out]
            n258 = call-poly <vilib>:"Write Key.vi"("section"=w415, "value"=w406, "key"="FrameRate", "refnum"=w417) -> ("refnum out"=w416:T20)  [unwired: 1 in, 6 out]
            n259 = property on="Camera Settings" class="Clust (strict)"("Visible"=w418) -> ()  [unwired: 2 in, 2 out]
            n260 = local write "DB Camera Config"(w418) -> ()
            n261 = call-poly <vilib>:"Write Key.vi"("section"=w415, "value"=w405, "key"="Compression", "refnum"=w416) -> ("refnum out"=w402:T20)  [unwired: 1 in, 6 out]
            n262 = call <vilib>:"Close Config Data.vi"("refnum"=w402) -> ("file path"=w403:path)  [unwired: 2 in, 8 out]
            n263 = call <vilib>:"Open Config Data.vi"("configuration file path"=w403) -> ("refnum"=w401:T20)  [unwired: 8 in, 2 out]
          }
          frame True {
            n264 = property on="Camera Settings" class="Clust (strict)"("Visible"=TRUE) -> ()  [unwired: 2 in, 2 out]
          }
        }
      }
      event "Camera Settings": Value Change {
        # "Update summary string when any elements of DB camera change"
        n265 = event-data() -> ("NewVal"=w433:T2)  [unwired: 1 in]
        n266 = Index Array(array=w429) -> (element=w428:cluster{string[]})  [unwired: 1 in]
        n267 = Unbundle(w433) -> ("Frame Rate"=w424:i32, "Compression"=w423:i32, "Size"=w426:u16)
        n268 = Unbundle(w428) -> (w427:string[])
        n269 = Index Array(array=w427, index=w426) -> (element=w425:string)
        n270 = Format Into String(format string="%s   %dfps   %d%%", w425, w424, w423) -> (resulting string=w430:string)  [unwired: 2 in, 1 out]
        n271 = Build Array(w430) -> (w431:string[])
        n272 = property on="DB Camera Config" class="Bool (strict)"("Strings [4]"=w431) -> ()  [unwired: 2 in, 2 out]
      }
      event "Motor.Enable": Value Change {
        # "When the test mode otor enable helper is set, update that\ntree row item's value"
        n273 = event-data() -> ("NewVal"=w440:bool)  [unwired: 1 in]
        n274 = Unbundle("Motor") -> ("Value"=w439:dbl)  [unwired: 1 out]
        n275 = Select(t=w439, s=w440, f=0.0) -> (s? t:f=w437:dbl)
        n276 = call <vilib>:"NT Write Number.vi"("Numeric"=w437, "Name"=w436) -> ()  [unwired: 9 in, 1 out]
      }
      event "Test Slider": Value Change {
        # "When the test mode slider helper is set, update that\ntree row item's value"
        n277 = event-data() -> ("NewVal"=w444:dbl)  [unwired: 1 in]
        n278 = call <vilib>:"NT Write Number.vi"("Numeric"=w444, "Name"=w445) -> ()  [unwired: 9 in, 1 out]
      }
      event "On/Off": Value Change {
        # "When the test mode on/off helper value is set, update that\ntree row item's value"
        n279 = event-data() -> ("NewVal"=w450:bool)  [unwired: 1 in]
        n280 = Boolean To (0,1)(Boolean=w450) -> (0, 1=w449:i16)
        n281 = call <vilib>:"NT Write Number.vi"("Numeric"=w449, "Name"=w448) -> ()  [unwired: 9 in, 1 out]
      }
      event "Rev/Fwd": Value Change {
        # "When the test mode helper value for relays is set, update that\ntree row item's value"
        n282 = event-data() -> ("NewVal.Forward"=w459:bool, "NewVal.Reverse"=w458:bool)  [unwired: 1 in]
        n283 = Boolean To (0,1)(Boolean=w459) -> (0, 1=w455:i16)
        n284 = Boolean To (0,1)(Boolean=w458) -> (0, 1=w457:i16)
        n285 = Negate(x=w457) -> (-x=w456:i16)
        n286 = Add(x=w455, y=w456) -> (x+y=w454:i16)
        n287 = call <vilib>:"NT Write Number.vi"("Numeric"=w454, "Name"=w453) -> ()  [unwired: 9 in, 1 out]
      }
      event "Test Ring": Value Change {
        # "When a test mode helper value is selected from the ring,\nset the tree item's variable to the string value"
        n288 = event-data() -> ("NewVal"=w464:u16)  [unwired: 1 in]
        n289 = property on="Test Ring" class="Ring (strict)"() -> ("Strings []"=w465:string[])  [unwired: 2 in, 2 out]
        n290 = Index Array(array=w465, index=w464) -> (element=w463:string)
        n291 = call <vilib>:"NT Write String.vi"("String"=w463, "Name"=w462) -> ()  [unwired: 9 in, 1 out]
      }
      event "Rec Mode": Value Change {
        # "Update globals for recording mode and path to read log from.\nClear when logging and let NetworkTables set path for vision to\nuse."
        n292 = event-data() -> ("NewVal"=w477:enum32{"Stop", "Record", "Playback"})  [unwired: 1 in]
        n293 = global write "WPI_DashboardLogging Global.vi" "Logging Filename"(path "") -> ()
        n294 = global write "WPI_DashboardLogging Global.vi" "Recording"(w477) -> ()
        n295 = case shown="\"Playback\"" w477 {
          tunnel: w476 -> [_ w479 w488]
          tunnel: [_ _ w487] -> w473
          tunnel: [_ _ w486] -> _
          tunnel: w471 -> [_ _ w484]
          tunnel: cluster{i32, i32} {-250, 170} -> [_ _ w483]
          tunnel: [_ _ T23 {"Image Size"=TRUE, "Image Type"=TRUE, "Pixel Value"=TRUE, "ROI Information"=TRUE, "Zoom Factor"=FALSE} ("Image Information Shown:All Elements")] -> w469
          tunnel: [_ _ TRUE ("Zoom Factor")] -> w468
          tunnel: w467 -> [_ _ w480]
          frame Default {
          }
          frame "Stop", "Record" {
            # "Place Window too"
            n296 = invoke class="VI" method="FP.Close"(reference=w479) -> (reference out=w478:refnum<vi>)  [unwired: 2 in, 2 out]
            n297 = invoke class="VI" method="Abort VI"(reference=w478) -> ()  [unwired: 2 in, 3 out]
          }
          frame "Playback" {
            n298 = call "Open Playback Panel.vi"("Offset"=w483, "DB VI Ref"=w484, "Playback in"=w488) -> ("Playback out"=w485:refnum<vi>)  [unwired: 8 in]
            n299 = register-events(w485, w480) -> (reference out=w487:refnum<event-registration>, error out=w486:errorcluster)  [unwired: 2 in]
          }
        }
        n300 = property on="Camera Image" class="ImageControl"("Image Information Shown"=w469, "Image Information Visible"=w468) -> ()  [unwired: 2 in, 2 out]
        n301 = call <vilib>:"WPI_DashboardNT Log FieldName Cache.vi"("Operation"=enum16{"Lookup/Add", "Index", "Clear"}."Clear") -> ()  [unwired: 8 in, 3 out]
      }
      event Panel Close {
        w490 = enum32{"Stop", "Record", "Playback"}."Stop" ("Rec Mode")
        # "Playback window has been closed, abort"
        n302 = event-data() -> ()  [unwired: 1 in, 4 out]
        n303 = local write "Rec Mode"(w490) -> ()
        n304 = global write "WPI_DashboardLogging Global.vi" "Recording"(w490) -> ()
      }
      event Panel Close {
        # "Abort playback window and ourself"
        n305 = event-data() -> ()  [unwired: 1 in, 4 out]
        n306 = invoke class="VI" method="FP.Close"(reference=w496) -> (reference out=w495:refnum<vi>)  [unwired: 2 in, 2 out]
        n307 = invoke class="VI" method="Abort VI"(reference=w495) -> (error out=w494:errorcluster)  [unwired: 2 in, 2 out]
        n308 = invoke class="VI" method="Abort VI"(error in=w494) -> ()  [unwired: 2 in, 3 out]
      }
      event User Event {
        n309 = event-data() -> ("IDs"=w504:cluster{"RPC field ID":u16, "Unique ID":u16}, "String"=w503:string)  [unwired: 1 in]
        n310 = Bundle("IDs"=w504, "String"=w503) -> (w502:T9)  [unwired: 1 in]
        n311 = call <vilib>:"Retrieve RPC Response.vi"("RPC Response"=w502) -> ("Output"=w499:string[][])  [unwired: 10 in]
        n312 = Build Array (concatenate)(w497, w499) -> (w498:string[][])
        n313 = local write "Command Params"(w498) -> ()
        n314 = local write "Cmd Status"("" ("Cmd Status")) -> ()
      }
      event "Vision": Value Change {
        # "Enable/Disable Compression slider.\nHW USB is hard-coded into the camera"
        n315 = event-data() -> ("NewVal"=w511:u16)  [unwired: 1 in]
        n316 = Equal?(x=w511, y=u32 2 ("milliseconds to wait")) -> (x = y?=w509:bool)
        n317 = Select(t=T24."Disabled and Grayed Out" ("Disabled"), s=w509, f=T24."Enabled" ("Disabled")) -> (s? t:f=w506:T24)
        n318 = property on="Compression" class="Slide (strict)"("DisabledEnum"=w506) -> ()  [unwired: 2 in, 2 out]
      }
      event "Tree": Double Click {
        n319 = event-data() -> ("PlatMods"=w516:T27, "Tag"=w515:string)  [unwired: 1 in]
        n320 = Unbundle(w516) -> ("Shift"=w514:bool)  [unwired: 4 out]
        n321 = Not(x=w514) -> (.not. x?=w513:bool)
        n322 = call <vilib>:"NT Update Persistence.vi"("Persistence"=w513, "Name"=w515) -> ()  [unwired: 9 in, 1 out]
      }
    }
  }
  n323 = while {
    tunnel: w47 -> [w520]
    i -> [w523]
    stop <- FALSE stop-if-true
    n324 = Wait (ms)(milliseconds to wait=u32 100) -> ()  [unwired: 1 out]
    n325 = case shown="\"Playback\"" "Rec Mode" {
      tunnel: w523 -> [_ _ w538]
      tunnel: [u32 2829099 ("Base Color") u32 11141120 ("Target Color") w527] -> w519
      frame "Stop", Default {
        # "Reset the color, extra updates don't cost much"
      }
      frame "Record" {
      }
      frame "Playback" {
        # "Playback"
        n326 = Quotient & Remainder(x=w538, y=u32 50 ("milliseconds to wait")) -> (x-y*floor(x/y)=w534:u32)  [unwired: 1 out]
        n327 = Divide(x=w534, y=u32 50 ("milliseconds to wait")) -> (x/y=w531:dbl)
        n328 = Multiply(x=6.283185307179586, y=w531) -> (x*y=w536:dbl)
        n329 = Sine(x=w536) -> (sin(x)=w535:dbl)
        n330 = Absolute Value(x=w535) -> (abs(x)=w528:dbl)
        n331 = call "Interpolate RGB Color.vi"("Proportion"=w528, "Target Color"=u32 30976, "Base Color"=u32 2829099) -> ("Result Color"=w527:u32)  [unwired: 8 in]
      }
    }
    n332 = property class="Pane"(reference=w520, "PaneColor"=w519) -> ()  [unwired: 1 in, 2 out]
  }
  n333 = local write "Dashboard Tab"(T1."Drive" ("Dashboard Tab")) -> ()
  n334 = property on="On/Off" class="Bool (strict)"("Visible"=w15) -> ()  [unwired: 2 in, 2 out]
  n335 = property on="Motor" class="Clust (strict)"("Visible"=w15) -> ()  [unwired: 2 in, 2 out]
  n336 = property on="Progress" class="Clust (strict)"("Visible"=w15) -> ()  [unwired: 2 in, 2 out]
  n337 = property on="Test Ring" class="Ring (strict)"("Visible"=w15) -> ()  [unwired: 2 in, 2 out]
  n338 = property on="Rev/Fwd" class="Clust (strict)"("Visible"=w15) -> ()  [unwired: 2 in, 2 out]
  n339 = property on="Camera Settings" class="Clust (strict)"("Visible"=w15) -> ()  [unwired: 2 in, 2 out]
  n340 = while {
    tunnel: u16 1741 ("timeout ms (25000)") -> [w540]
    stop <- FALSE stop-if-true
    n341 = TCP Create Listener(10:w540) -> (0:w539:errorcluster, 3:w541:refnum<k5>)  [unwired: 4 in, 1 out]
    n342 = case shown="No Error" w539 {
      selector: w539 -> [w543 _]
      tunnel: w541 -> [w544 _]
      frame No Error {
        n343 = while {
          tunnel: w544 -> [w547]
          tunnel: w543 -> [w546]
          stop <- FALSE stop-if-true
          n344 = TCP Wait On Listener(8:w546, 11:w547) -> (0:w548:errorcluster, 4:w549:refnum<k5>)  [unwired: 2 in, 3 out]
          n345 = local write "TCP"(w549) -> ()
          n346 = case shown="No Error" w548 {
            frame No Error {
            }
            frame Error {
              n347 = Wait (ms)(milliseconds to wait=u32 1000) -> ()  [unwired: 1 out]
            }
          }
        }
      }
      frame Error {
        n348 = Wait (ms)(milliseconds to wait=u32 1000) -> ()  [unwired: 1 out]
      }
    }
  }
  n349 = local write "DB Camera Config"(w15) -> ()
  n350 = local write "Command Params"(string[][] [] ("Command Params")) -> ()
  n351 = global write "WPI_DashboardLogging Global.vi" "Recording"(w41) -> ()
  n352 = local write "Command Selection"(u16 0 ("milliseconds to wait")) -> ()
  n353 = local write "Rec Mode"(w41) -> ()
